vi "ReadProjectNode.vi"(8 "Error In":errorcluster, 11 "Experiment Node In":refnum<k20>) -> (0 "Error Out":errorcluster, 2 "Project":string, 3 "Experiment Node Out":refnum<k20>)   [LabVIEW 2012]
uses:
  <vilib>/xml/NI_XML.lvlib
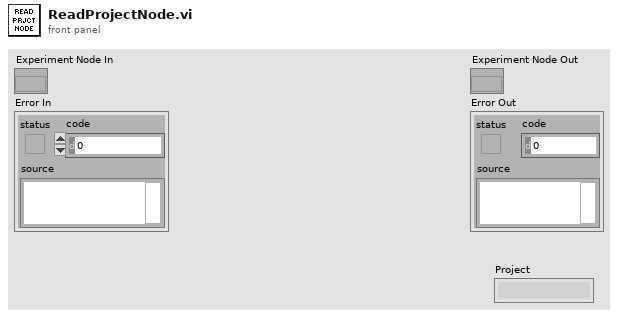
[diagram p1: front panel]
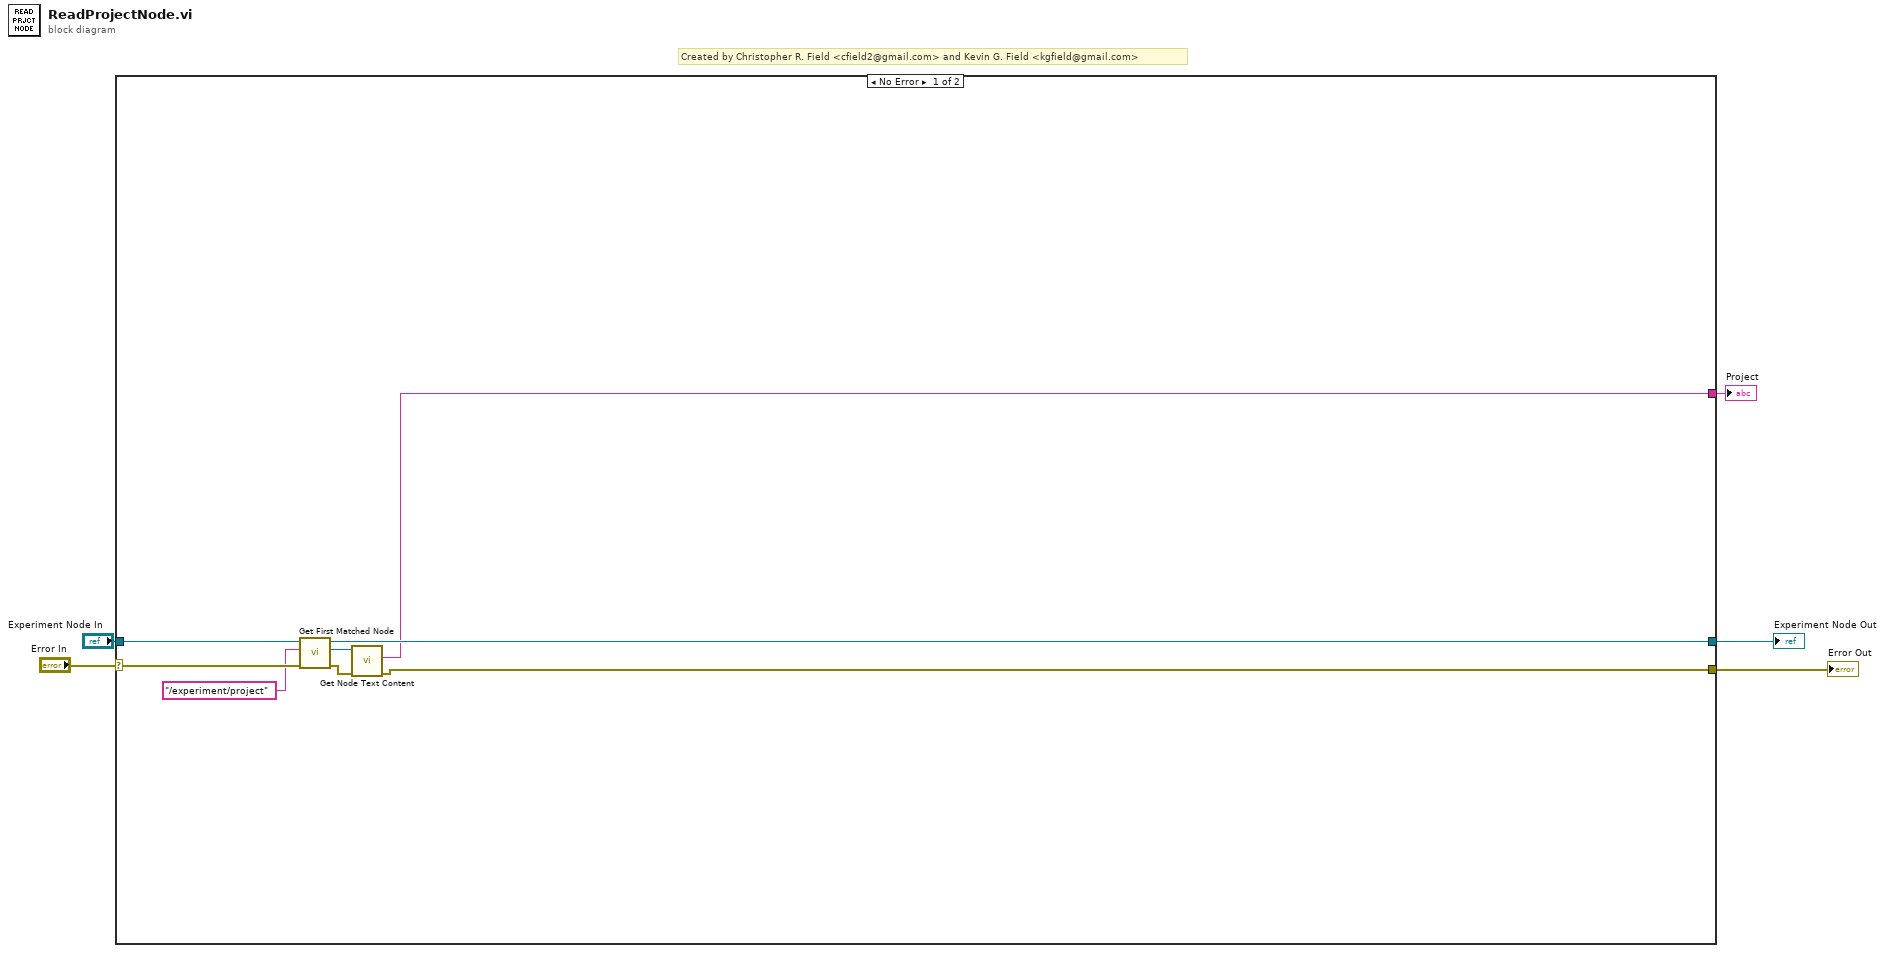
[diagram p0: block diagram]
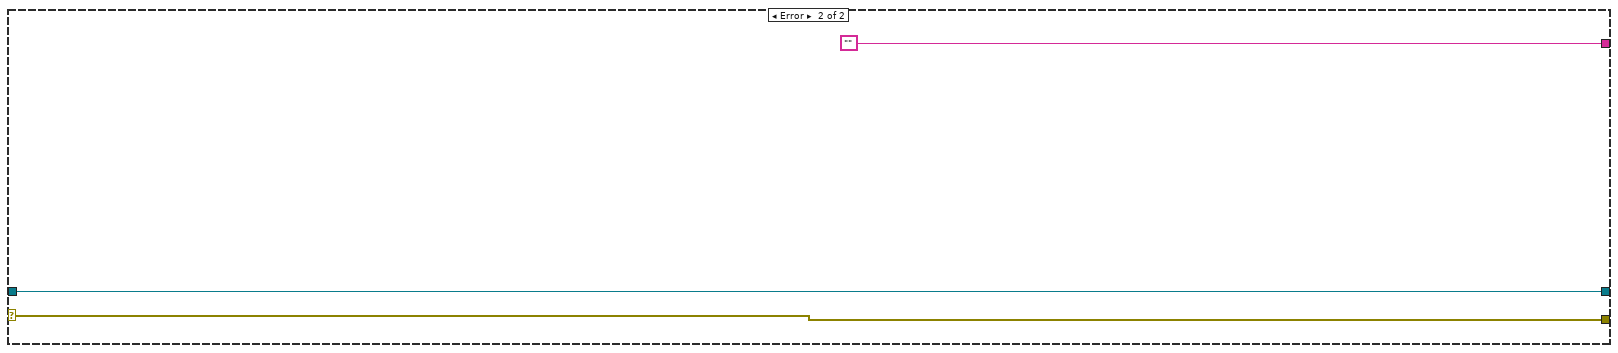
[diagram p2: hidden frame]
diagram:
  # "Created by Christopher R. Field <cfield2@gmail.com> and Kevin G. Field <kgfield@gmail.com>"
  n1 = case shown="No Error" "Error In" {
    selector: "Error In" -> [w12 w15]
    tunnel: "Experiment Node In" -> [w13 w16]
    tunnel: [w8 w16] -> w3
    tunnel: [w7 w15] -> w2
    tunnel: [w6 ""] -> w1
    frame No Error {
      n2 = call <vilib>:"Get First Matched Node.vi"("error in (no error)"=w12, "XPath expression"="/experiment/project", "node in"=w13) -> ("error out"=w9:errorcluster, "node result"=w10:refnum<k20>, "node out"=w8:refnum<k20>)  [unwired: 6 in]
      n3 = call <vilib>:"Get Node Text Content.vi"("error in (no error)"=w9, "node in"=w10) -> ("error out"=w7:errorcluster, "node text"=w6:string)  [unwired: 7 in, 1 out]
    }
    frame Error {
    }
  }
  "Experiment Node Out" <- w3
  "Error Out" <- w2
  "Project" <- w1
